vi "ConfigurationsControlLoop.vi"   [LabVIEW 2016]
uses:
  Configurations.vi
  <vilib>/Rock Robotics/Network Tables/NT Read Boolean.vi
types:
  T1 = enum16{"open", "replace", "create", "open or create", "replace or create", "replace or create with confirmation"}
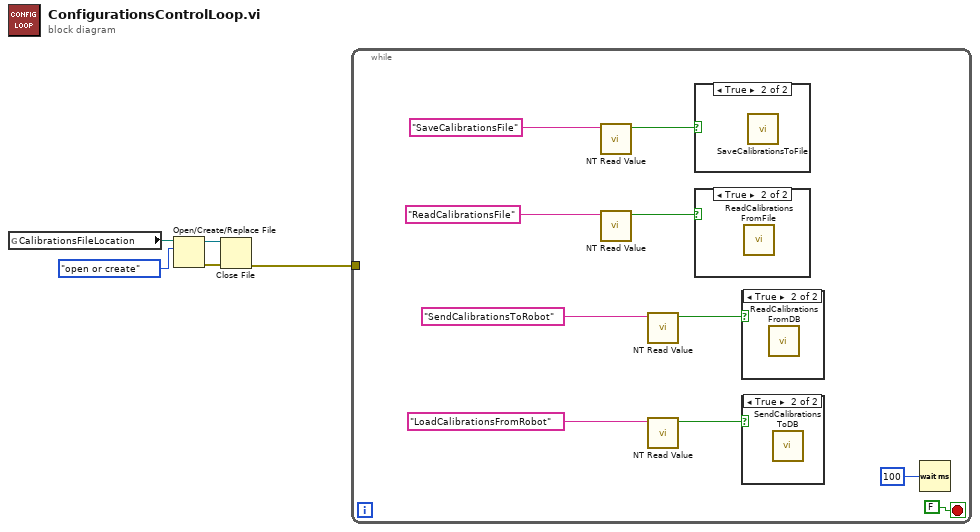
[diagram p0: block diagram]
diagram:
  n1 = global read "Configurations.vi" "CalibrationsFileLocation"() -> (w5:path)
  n2 = Open/Create/Replace File(file path (use dialog)=w5, operation (0:open)=T1."open or create") -> (refnum out=w3:refnum<file>, error out=w2:errorcluster)  [unwired: 4 in, 1 out]
  n3 = Close File(refnum=w3, error in=w2) -> (error out=w1:errorcluster)  [unwired: 1 out]
  n4 = while {
    tunnel: w1 -> [_]
    stop <- FALSE stop-if-true
    n5 = call-poly <vilib>:"NT Read Value.vi"("Name"="SaveCalibrationsFile") -> ("Boolean"=w8:bool)  [unwired: 9 in, 1 out]
    n6 = call-poly <vilib>:"NT Read Value.vi"("Name"="ReadCalibrationsFile") -> ("Boolean"=w6:bool)  [unwired: 9 in, 1 out]
    n7 = call-poly <vilib>:"NT Read Value.vi"("Name"="SendCalibrationsToRobot") -> ("Boolean"=w12:bool)  [unwired: 9 in, 1 out]
    n8 = call-poly <vilib>:"NT Read Value.vi"("Name"="LoadCalibrationsFromRobot") -> ("Boolean"=w11:bool)  [unwired: 9 in, 1 out]
    n9 = case shown="True" w8 {
      frame False {
      }
      frame True {
        n10 = call "SaveCalibrationsToFile.vi"() -> ()  [unwired: 12 in]
      }
    }
    n11 = case shown="True" w6 {
      frame False {
      }
      frame True {
        n12 = call "ReadCalibrationsFromFile.vi"() -> ()  [unwired: 12 in]
      }
    }
    n13 = case shown="True" w12 {
      frame False {
      }
      frame True {
        n14 = call "ReadCalibrationsFromDB.vi"() -> ()  [unwired: 12 in]
      }
    }
    n15 = case shown="True" w11 {
      frame False {
      }
      frame True {
        n16 = call "SendCalibrationsToDB.vi"() -> ()  [unwired: 12 in]
      }
    }
    n17 = Wait (ms)(milliseconds to wait=u32 100) -> ()  [unwired: 1 out]
  }
